vi "My Custom Controls - Graph with Tare Recording.vi"() -> ()   [LabVIEW 2016]
doc: "Sample numeric display item."
uses:
  <vilib>/NI Veristand/Display Template Support/Display Template Support.llb/enum_Graph Handler Message.ctl
  <vilib>/NI Veristand/Display Template Support/Display Template Support.llb/cluster_Graph Handler Message.ctl
  <vilib>/NI Veristand/Display Template Support/Display Template Support.llb/sub_Display Template Handler Graph.vi
  <vilib>/NI Veristand/Display Template Support/Display Template Support.llb/sub_Display Template Data Handler Graph.vi
  _subVIs/Message Queue/Message Queue.lvlib
  _subVIs/User Event - Stop/User Event - Stop.lvlib
  _subVIs/Message Queue/Enqueue Message (Single).vi
  <vilib>/NI Veristand/Display Template Support/Display Template Support.llb/cluster_Screen Item Settings.ctl
  <vilib>/NI Veristand/Display Template Support/Display Template Support.llb/cluster_Graph Scale Settings.ctl
  <vilib>/NI Veristand/Display Template Support/Display Template Support.llb/cluster_Graph Plot Settings.ctl
panel:
  out "appended path":path
  in  "NIVS.Project File Path":path
  out "data":u32
  out "Record command count":i32
  out "Wait.Time":u32
  out "Graph":waveform(dbl)[](graph)
  out "Label":string="Numeric"
  out "Value Stored":dbl
  in  "Store Value":bool
  in  "Plot Index":dbl
  out "Data Lost":bool
  out "Y.Autoscale":bool
  in  "Y.Scale.Once":bool
  in  "Y.Scale.Auto":bool
  out "X.Autoscale":bool
  in  "X.Scale.Once":bool
  in  "X.Scale.Auto":bool
  in  "Legend":bool
  in  "Setup":bool
  in  "Hold":bool
  in  "Item.Data":T1
  # "Autoscale X"
  # "Autoscale Y"
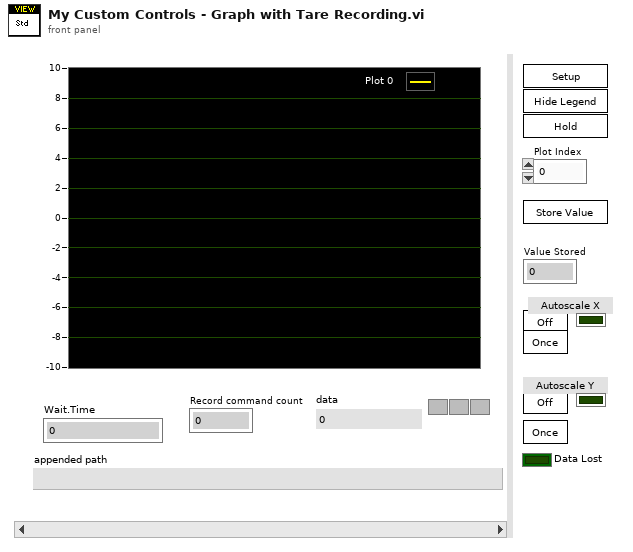
[diagram p1: front panel]
types:
  T1 = typedef "cluster_Screen Item Settings.ctl" = cluster{"Template VI":string, "Position X":i32, "Position Y":i32, "Custom":string, "Show Title Bar":bool, "ID":i32, "Always On Top":bool, "Allow Resize":bool, "Allow Minimize":bool, "Allow Close":bool, "Size to Screen":bool, "Screen.ID":i32, "State":enum16{"Normal", "New"}, "Title":string, "Window Bounds":cluster{"[0]":i16, "[1]":i16, "[2]":i16, "[3]":i16}, "Channel Ref":u64, "Unit":string, "Default Units?":bool, "Flash Limit?":bool, "Color 1":u32, "Color 2":u32, "Color 3":u32, "Color 4":u32, "Bck Color":u32, "Fore Color":u32, "Limit 1":dbl, "Limit 2":dbl, "Limit 3":dbl, "Limit 4":dbl, "Limit Mode 1":i32, "Limit Mode 2":i32, "Limit Mode 3":i32, "Limit Mode 4":i32, "Scale Precision":i32, "Scale Min":dbl, "Scale Max":dbl, "Format":i32, "Precision":i32, "Background Type":i32, "IDs":i32[], "Units":string[], "Labels":string[], "Scale Factor":dbl, "Scale Offset":dbl, "YScale Index":u32[], "XScale":T2, "YScales":T2[], "Plots":T3[], "Update Period":dbl, "History Length":dbl, "My.Ref":refnum<vi>, "Is Control?":bool, "Channel Paths":string[], "Custom Data":variant}
  T2 = typedef "cluster_Graph Scale Settings.ctl" = cluster{"Format":u8, "Precision":u8, "Fit":u8, "Label":string, "Use Default Label":bool, "Label Visible":bool, "Min":dbl, "Max":dbl}
  T3 = typedef "cluster_Graph Plot Settings.ctl" = cluster{"Bar Style":u8, "Fill To":i16, "Fill/PtColor":u32, "Line Style":u8, "Line Width":u8, "Color":u32, "Interp":u8, "Point Style":u8}
  T4 = typedef "cluster_Graph Handler Message.ctl" = cluster{"Message":T5, "Data":variant}
  T5 = typedef "enum_Graph Handler Message.ctl" = enum16{"None", "Stop", "Hold", "Update Channels", "New Settings", "Control Value", "Edit Value"}
  T6 = typedef "Message Queue.lvlib/All Message Queues.ctl" = cluster{"UI":refnum<queue>}
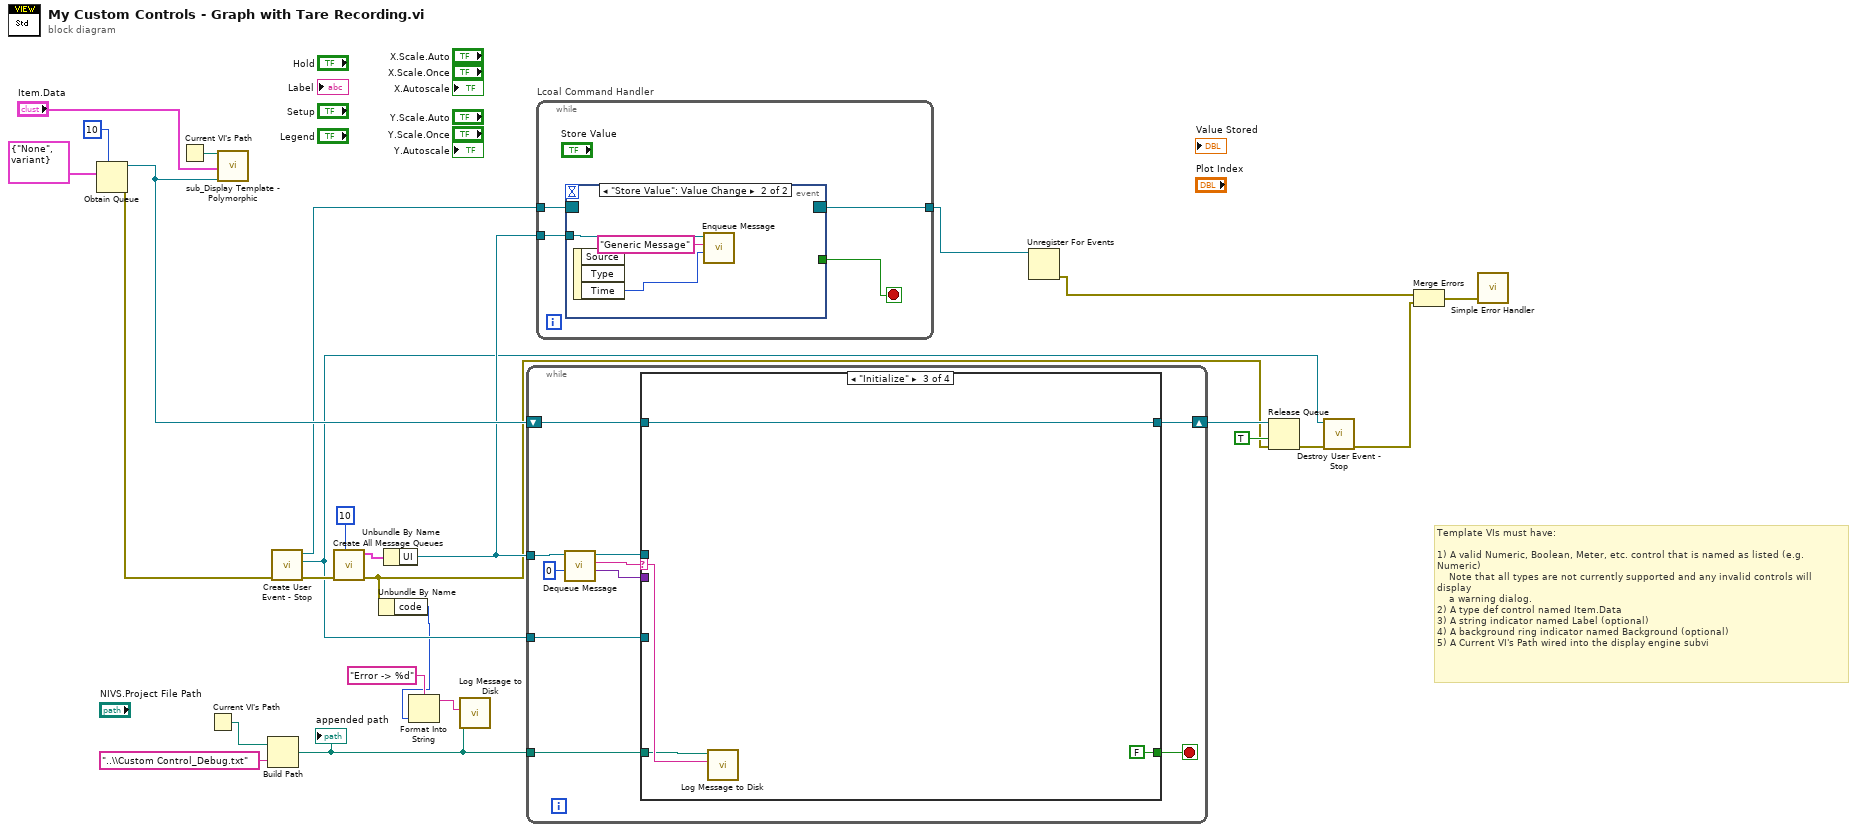
[diagram p0: block diagram]
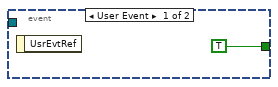
[diagram p2: hidden frame]
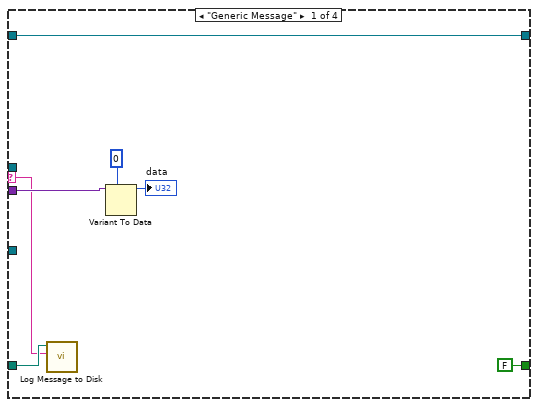
[diagram p3: hidden frame]
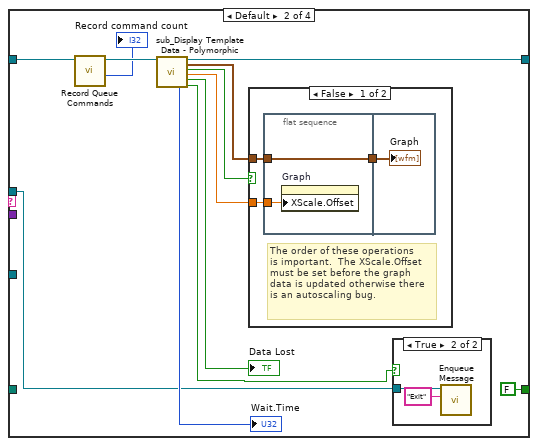
[diagram p4: hidden frame]
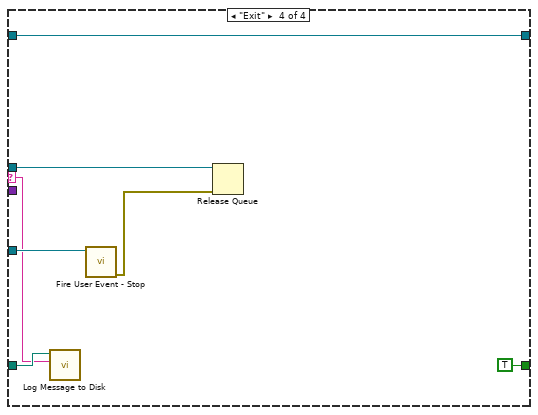
[diagram p7: hidden frame]
diagram:
  # "Template VIs must have:\n\n1) A valid Numeric, Boolean, Meter, etc. control that is named as listed (e.g. Numeric)\n    Note that all types are not currently supported and any invalid controls will display\n    a warning dialog.\n2) A type def control named Item.Data\n3) A string indicator named Label (optional)\n4) A background ring indicator named Background (optional)\n5) A Current VI's Path wired into the display engine subvi"
  n1 = Obtain Queue(max queue size (-1, unlimited)=10, element data type=T4 {"Message"=enum."None", "Data"=variant} ("Message")) -> (queue out=w20:refnum<queue>, error out=w4:errorcluster)  [unwired: 2 in, 2 out]
  n2 = Current VI's Path() -> (path=w26:path)
  n3 = Current VI's Path() -> (path=w1:path)
  n4 = call-poly <vilib>:"sub_Display Template - Polymorphic.vi"("Parent.Path"=w26, "Item.Data"="Item.Data", "queue"=w20) -> ()  [unwired: 17 out]
  n5 = Build Path(base path=w1, name or relative path="..\\Custom Control_Debug.txt") -> (appended path=w2:path)
  "appended path" <- w2
  n6 = call "Create User Event - Stop.vi"("error in (no error)"=w4) -> ("error out"=w18:errorcluster, "User Event - Stop"=w14:refnum<user-event>, "Stop Event Registration Refnum"=w17:refnum<event-registration>)  [unwired: 8 in]
  n7 = call "Create All Message Queues.vi"("max queue size (-1, unlimited)"=10, "error in (no error)"=w18) -> ("error out"=w9:errorcluster, "Message Queues out"=w16:T6)  [unwired: 8 in]
  n8 = Unbundle By Name(w9) -> ("code"=w7:i32)
  n9 = Unbundle By Name(w16) -> ("UI"=w19:refnum<queue>)
  n10 = Format Into String(format string="Error -> %d", w7) -> (resulting string=w6:string)  [unwired: 2 in, 1 out]
  n11 = call <userlib>:"Log Message to Disk.vi"("Message"=w6, "Log File Path (FM_debug.txt)"=w2) -> ()  [unwired: 9 in, 1 out]
  n12 = while {
    shift-right: [w36] -> w24
    shift-left: w20 -> [w34]
    tunnel: w19 -> [w33]
    tunnel: w14 -> [w29]
    tunnel: w2 -> [w27]
    stop <- w35 stop-if-true
    n13 = call "Dequeue Message.vi"("timeout in ms (0)"=0, "Message Queue"=w33) -> ("Message Data"=w31:variant, "Message"=w28:string, "dup Message Queue"=w30:refnum<queue>)  [unwired: 5 in, 2 out]
    n14 = case shown="\"Initialize\"" w28 {
      selector: w28 -> [w37 _ w65 w68]
      tunnel: [w40 w55 w67 w74] -> w36
      tunnel: [FALSE ("Stop") FALSE ("Stop") FALSE ("Stop") TRUE ("Stop")] -> w35
      tunnel: w34 -> [w40 w49 w67 w74]
      tunnel: w31 -> [w43 _ _ _]
      tunnel: w30 -> [_ w46 _ w72]
      tunnel: w29 -> [_ _ _ w73]
      tunnel: w27 -> [w38 _ w64 w69]
      frame "Generic Message" {
        n15 = call <userlib>:"Log Message to Disk.vi"("Message"=w37, "Log File Path (FM_debug.txt)"=w38) -> ()  [unwired: 9 in, 1 out]
        n16 = Variant To Data(type=u32 0 ("Time"), Variant=w43) -> (data=→"data":u32)  [unwired: 1 in, 1 out]
      }
      frame Default {
        n17 = call "Record Queue Commands.vi"("queue In"=w49) -> ("Record command count"=→"Record command count":i32, "queue Out"=w48:refnum<queue>)  [unwired: 7 in, 2 out]
        n18 = call-poly <vilib>:"sub_Display Template Data - Polymorphic.vi"("queue"=w48) -> ("Wait.Time"=→"Wait.Time":u32, "queue out"=w55:refnum<queue>, "Graph.Data"=w54:waveform(dbl)[], "Hold"=w52:bool, "XScale.Offset"=w53:dbl, "Data Lost"=→"Data Lost":bool, "Stop"=w45:bool)  [unwired: 12 out]
        n19 = case shown="False" w52 {
          tunnel: w53 -> [w60 _]
          tunnel: w54 -> [w59 _]
          frame False {
            # "The order of these operations\nis important.  The XScale.Offset\nmust be set before the graph\ndata is updated otherwise there\nis an autoscaling bug."
            n20 = flat-sequence {
              tunnel: w60 -> [w62]
              tunnel: w59 -> [w61]
              tunnel: [w61] -> w58
              tunnel: w58 -> [w63]
              frame #0 {
                n21 = property on="Graph" class="WFGraph (strict)"("XScale.Offset"=w62) -> ()  [unwired: 2 in, 2 out]
              }
              frame #1 {
                "Graph" <- w63
              }
            }
          }
          frame True {
          }
        }
        n22 = case shown="True" w45 {
          tunnel: w46 -> [_ w57]
          frame False {
          }
          frame True {
            n23 = call-poly "Enqueue Message.vi"("Message"="Exit", "Message Queue"=w57) -> ()  [unwired: 8 in, 2 out]
          }
        }
      }
      frame "Initialize" {
        n24 = call <userlib>:"Log Message to Disk.vi"("Message"=w65, "Log File Path (FM_debug.txt)"=w64) -> ()  [unwired: 9 in, 1 out]
      }
      frame "Exit" {
        n25 = call <userlib>:"Log Message to Disk.vi"("Message"=w68, "Log File Path (FM_debug.txt)"=w69) -> ()  [unwired: 9 in, 1 out]
        n26 = call "Fire User Event - Stop.vi"("User Event - Stop"=w73) -> ("error out"=w71:errorcluster)  [unwired: 10 in]
        n27 = Release Queue(queue=w72, error in (no error)=w71) -> ()  [unwired: 1 in, 3 out]
      }
    }
  }
  n28 = while "Lcoal Command Handler" {
    tunnel: w19 -> [w77]
    tunnel: w17 -> [w78]
    tunnel: [w76] -> w5
    stop <- w75 stop-if-true
    n29 = event shown="[1] \"Store Value\": Value Change" {
      selector: w78 -> [_ _]
      dyn-events: [_ _] -> w76
      timeout: _ -> [_ _]
      tunnel: w77 -> [_ w82]
      tunnel: [TRUE _] -> w75
      event User Event {
        n30 = event-data() -> ()  [unwired: 1 in, 1 out]
      }
      event "Store Value": Value Change {
        n31 = event-data() -> ("Time"=w80:u32)  [unwired: 1 in, 2 out]
        n32 = call-poly "Enqueue Message.vi"("Message Data"=w80, "Message"="Generic Message", "Message Queue"=w82) -> ()  [unwired: 7 in, 2 out]
      }
    }
  }
  n33 = Unregister For Events(event registration refnum=w5) -> (error out=w13:errorcluster)  [unwired: 1 in]
  n34 = Release Queue(queue=w24, force destroy? (F)=TRUE, error in (no error)=w9) -> (error out=w15:errorcluster)  [unwired: 2 out]
  n35 = call "Destroy User Event - Stop.vi"("error in (no error)"=w15, "User Event - Stop"=w14) -> ("error out"=w12:errorcluster)  [unwired: 9 in]
  n36 = Merge Errors(w13, w12) -> (w11:errorcluster)
  n37 = call <vilib>:"Simple Error Handler.vi"("error in (no error)"=w11) -> ()  [unwired: 4 in, 5 out]
